vi "Dashboard Main.vi"() -> ()   [LabVIEW 2015]
uses:
  <vilib>/Utility/miscctls.llb/LVRowAndColumnTypeDef.ctl
  <vilib>/event_ctls.llb/eventvkey.ctl
  <vilib>/Rock Robotics/WPI/Dashboard/WPI_DashboardLogging Global.vi
  <vilib>/Rock Robotics/Network Tables/NT Read Numeric Array.vi
  <vilib>/Rock Robotics/Network Tables/NT Write Boolean Array.vi
  <vilib>/Rock Robotics/Network Tables/NT Write Numeric Array.vi
  <vilib>/Rock Robotics/Network Tables/NT Read Boolean Array.vi
  <vilib>/Rock Robotics/Network Tables/NT Write Boolean.vi
  <vilib>/Utility/config.llb/Write Key (String).vi
  <vilib>/Utility/config.llb/Write Key (I32).vi
  <vilib>/Utility/config.llb/NI_LVConfig.lvlib
panel:
  in  "TCP":refnum<k5>
  out "Camera IP":string
  out "Image Message":string="Timeout in Camera Communications"
  in  "Dashboard Tab":T1(tab)
  in  "Select Auto":string(combo)
  out "NT Connection":bool
  in  "Camera Settings":T2={"Frame Rate"=30, "Compression"=30, "Size"=1} {"Frame Rate" scale=1.0..30.0; "Size" items=["640x480", "320x240", "160x120"]}
  out "MotorChart R":cluster{"Numeric":dbl, "Numeric":dbl}(graph)
  out "MotorChart L":T3(graph)
  out "MotorSliders R":cluster{"MotorSlide1":dbl, "MotorSlide2":dbl} {"MotorSlide2" scale=-1.0..1.0 scale format="%#_2e"; "MotorSlide1" scale=-1.0..1.0 scale format="%#_2e"}
  out "MotorSliders L":T4 {"MotorSlide4 2" scale=0.0..14.0 scale format="%#_2e"; "MotorSlide2" scale=-1.0..1.0 scale format="%#_2e"; "MotorSlide1" scale=-1.0..1.0 scale format="%#_2e"}
  out "Gyro":dbl(knob) scale=0.0..360.0
  out "JS1 Z":dbl(slide) scale=-1.0..1.0 scale format="%#_2e"
  out "JS1 Graph":cluster{"X":dbl, "Y":dbl}[](graph)
  out "JS1 Buttons":T5
  out "JS2 Z":dbl(slide) scale=-1.0..1.0 scale format="%#_2e"
  out "JS2 Graph":cluster{"X":dbl, "Y":dbl}[](graph)
  out "JS2 Buttons":T5
  out "Mode":T6(ring)=enum."Auto Disabled"
  in  "DB Camera Config":bool
  out "fps":dbl format="%#.1g"
  out "Mbps":dbl format="%#.1g"
  out "Mbps LED":bool
  in  "Vision":u16(ring) items=["Camera Off", "USB Camera SW", "USB Camera HW", "IP Camera"]
  in  "Rec Mode":enum32{"Stop", "Record", "Playback"}(radio)
  out "Analogue 3":dbl
  out "Analogue 2":dbl
  out "Analogue 1":dbl
  out "Analogue 0":dbl
  in  "SOLENOID 7":bool
  in  "SOLENOID 6":bool
  in  "SOLENOID 5":bool
  in  "SOLENOID 4":bool
  in  "SOLENOID 3":bool
  in  "SOLENOID 2":bool
  in  "SOLENOID 1":bool
  in  "SOLENOID 0":bool
  in  "Compressor":bool
  in  "RELAY 3":enum16{"Off", "On", "Forward", "Reverse"}(ring)
  in  "RELAY 2":enum16{"Off", "On", "Forward", "Reverse"}(ring)
  in  "RELAY 1":enum16{"Off", "On", "Forward", "Reverse"}(ring)
  in  "RELAY 0":enum16{"Off", "On", "Forward", "Reverse"}(ring)
  out "DIO 9":bool
  out "DIO 8":bool
  out "DIO 7":bool
  out "DIO 6":bool
  out "DIO 5":bool
  out "DIO 4":bool
  out "DIO 3":bool
  out "DIO 2":bool
  out "DIO 1":bool
  out "DIO 0":bool
  in  "Motor 2 Controller":T7(radio)
  in  "Invert Motor 2":bool
  out "Current Motor 2 Type":string
  in  "Select Motor 2 Address":dbl
  in  "Select Motor 2 Type":u16(ring)=101 items=["CAN Jaguar"=0, "Jaguar"=1, "CAN Talon"=2, "Talon (SR)"=3, "Talon SRX"=4, "Victor"=5, "Victor SP"=6, "Null"=101]
  in  "Motor 1 Controller":T7(radio)
  in  "Invert Motor 1":bool
  out "Current Motor 1 Type":string
  in  "Select Motor 1 Address":dbl
  in  "Select Motor 1 Type":u16(ring)=101 items=["CAN Jaguar"=0, "Jaguar"=1, "CAN Talon"=2, "Talon (SR)"=3, "Talon SRX"=4, "Victor"=5, "Victor SP"=6, "Null"=101]
  out "Motor 1":dbl(knob) scale=-1.0..1.0
  in  "Set Motor":bool
  in  "Joystick Deadband":dbl=0.2
  out "Motor 2":dbl(knob) scale=-1.0..1.0
  in  "Test Slider":dbl(slide) scale=0.0..100.0 scale format="%#_3g"
  in  "On/Off":bool caption="Solenoid"
  in  "Test Name":u16(ring) items=["Select the test to run..."]
  in  "Test Tree":string(tree)
  in  "Motor":cluster{"Value":dbl, "Enable":bool} {"Value" scale=-1.0..1.0 scale format="%#_3g"}
  out "Progress":T8 {"Test Progress" scale=0.0..100.0}
  in  "Rev/Fwd":cluster{"Forward":bool, "Reverse":bool}
  in  "Test Ring":u16(ring) items=["Monochrome", "Color"]
  out "Cmd Status":string
  in  "Execute Command":bool
  in  "Command Params":string[][](table)
  in  "Command Selection":i32(listbox)
  in  "CheckList":i32(listbox)
  out "Tree":string(tree)
  out "Camera Image":T9(plugin-control)
  out "Background":bool
  # "Left"
  # "Front"
  # "Right"
  # "Battery"
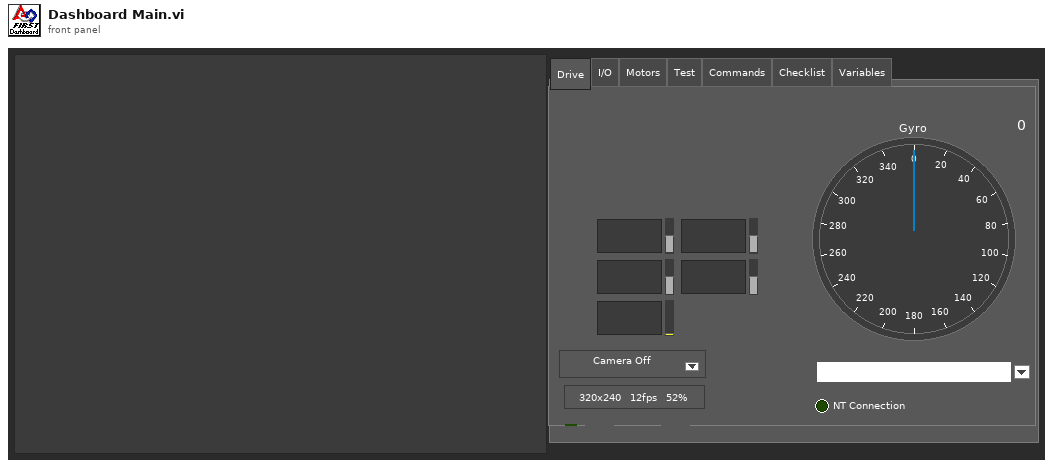
[diagram p1: front panel]
types:
  T1 = enum32{"Drive", "I/O", "Motors", "Test", "Commands", "Checklist", "Variables"}
  T2 = cluster{"Frame Rate":i32, "Compression":i32, "Size":u16}
  T3 = cluster{"Numeric":dbl, "Numeric":dbl, "Battery V":dbl}
  T4 = cluster{"MotorSlide1":dbl, "MotorSlide2":dbl, "MotorSlide4 2":dbl}
  T5 = cluster{bool, bool, bool, bool, bool, bool, bool, bool, bool, bool, bool, bool}
  T6 = enum8{"Tele-Op Disabled", "Tele-Op Enabled", "Auto Disabled", "Auto Enabled", "Test Disabled", "Test Enabled", "Disconnected", "No Code", "E-Stop"}
  T7 = enum32{"Radio Selection 1", "Radio Selection 2", "Radio Selection 3"}
  T8 = cluster{"Test Progress":u8, "Test Progress Text":string}
  T9 = typedef "IMAQ Image.ctl" = refnum<image>
  T10 = cluster{"IDs":cluster{"RPC field ID":u16, "Unique ID":u16}, "String":string}
  T11 = enum32{"Drive", "Basic", "Custom", "Test", "Checklist", "Variables"}
  T12 = typedef "Image Type" = u32
  T13 = cluster{"Camera Image":refnum<vi>, "Dashboard Tab":refnum<vi>, "Background":refnum<vi>, "Vision":refnum<vi>, "Rec Mode":refnum<vi>, "Test Slider":refnum<vi>, "On/Off ":refnum<vi>, "Test Ring":refnum<vi>, "Rev/Fwd":refnum<vi>, "Test Name":refnum<vi>, "Motor":refnum<vi>, "Progress":refnum<vi>, "CheckList":refnum<vi>, "Tree":refnum<vi>, "Test Tree":refnum<vi>, "Command Params":refnum<vi>, "Command Selection":refnum<vi>, "Execute Command":refnum<vi>, "Cmd Status":refnum<vi>}
  T14 = cluster{"Error Strings":string, "Disable Counts":cluster{u16, u16}, "Rail Faults":cluster{u16, u16, u16}, "Robot IP":string, "DB Mode":u8, "Event Info":cluster{"Name":string, "Type":u8, "Number":u16, "Replay":u8}, "Camera Addr":string}
  T15 = cluster{"Storage":cluster{"Disk Free":u64, "RAM Block":u32, "RAM free":u32}, "CPU Utilization":cluster{"CPU % ISR":sgl, "CPU % Time Crit":sgl, "CPU % Timed Str":sgl, "CPU % High":sgl, "CPU % Above":sgl, "CPU % Normal":sgl, "CPU % Low":sgl}, "CAN":cluster{"% Bus Utilization":sgl, "Bus Off Cnt":u32, "TX_FIFO Full Cnt":u32, "Receive Error Cnt":u8, "Transmit Error Cnt":u8}, "HID":cluster{"HID Outputs":u32, "Rumble Low":u16, "Rumble High":u16}[]}
  T16 = cluster{"Status bits":cluster{"Test Mode":bool, "Autonomous":bool, "Enabled":bool, "Code Start":bool, "Brownout":bool, "Reserved 2":bool, "Reserved 3":bool, "E-Stop":bool}, "Code Trace":cluster{"Disabled":bool, "TeleOp":bool, "Auto":bool, "Test":bool}, "Controller Type":enum16{"unknown", "cRIO", "roboRio"}, "Code?":enum16{"unknown", "noCode", "code"}, "Battery V":dbl}
  T17 = cluster{"Control Bits":cluster{"TestMode":bool, "Autonomous":bool, "Enabled":bool, "FMS Present":bool, bool, bool, bool, "E-Stop":bool}, "Team Station ":u8, "Countdown":sgl, "Joystick Values":cluster{"Axes":dbl[], "Buttons":bool[], "POVs":i16[]}[]}
  T18 = cluster{"Axes":dbl[], "Buttons":bool[], "POVs":i16[]}[]
  T19 = cluster{"Axes":dbl[], "Buttons":bool[], "POVs":i16[]}
  T20 = cluster{"Buttons[0]":bool, "Buttons[1]":bool, "Buttons[2]":bool, "Buttons[3]":bool, "Buttons[4]":bool, "Buttons[5]":bool, "Buttons[6]":bool, "Buttons[7]":bool, "Buttons[8]":bool, "Buttons[9]":bool, "Buttons[10]":bool, "Buttons[11]":bool}
  T21 = typedef "NI_LVConfig.lvlib/Config Data RefNum.ctl" = refnum<k1>
  T22 = cluster{"Operation":enum16{"Update", "Clear"}, "Color Box":u32}[]
  T23 = typedef "eventvkey.ctl" = enum16{"ASCII", "Enter", "Return", "Shift", "Ctrl", "Alt", "Cmd", "Opt", "Caps", "NumLock", "Clear", "Break", "Up", "Down", "Left", "Right", "Insert", "Delete", "Home", "End", "PageUp", "PageDown", "Escape", "Help", "Pause", "ScrollLock", "F1", "F2", "F3", "F4", "F5", "F6", "F7", "F8", "F9", "F10", "F11", "F12", "F13", "F14", "F15", "F16", "F17", "F18", "F19", "F20", "F21", "F22", "F23", "F24", "Play", "VolumeUp", "VolumeDown", "Mute", "Two Byte Char"}
  T24 = cluster{"Image Size":bool, "Image Type":bool, "Pixel Value":bool, "ROI Information":bool, "Zoom Factor":bool}
  T25 = enum8{"Enabled", "Disabled", "Disabled and Grayed Out"}
  T26 = cluster{"Operation":enum16{"Update", "Clear"}, "Color Box":u32}
  T27 = typedef "LVRowAndColumnTypeDef.ctl" = cluster{"Row":i32, "Column":i32}
  T28 = cluster{"Shift":bool, "Ctrl":bool, "Alt":bool, "Cmd":bool, "Opt":bool}
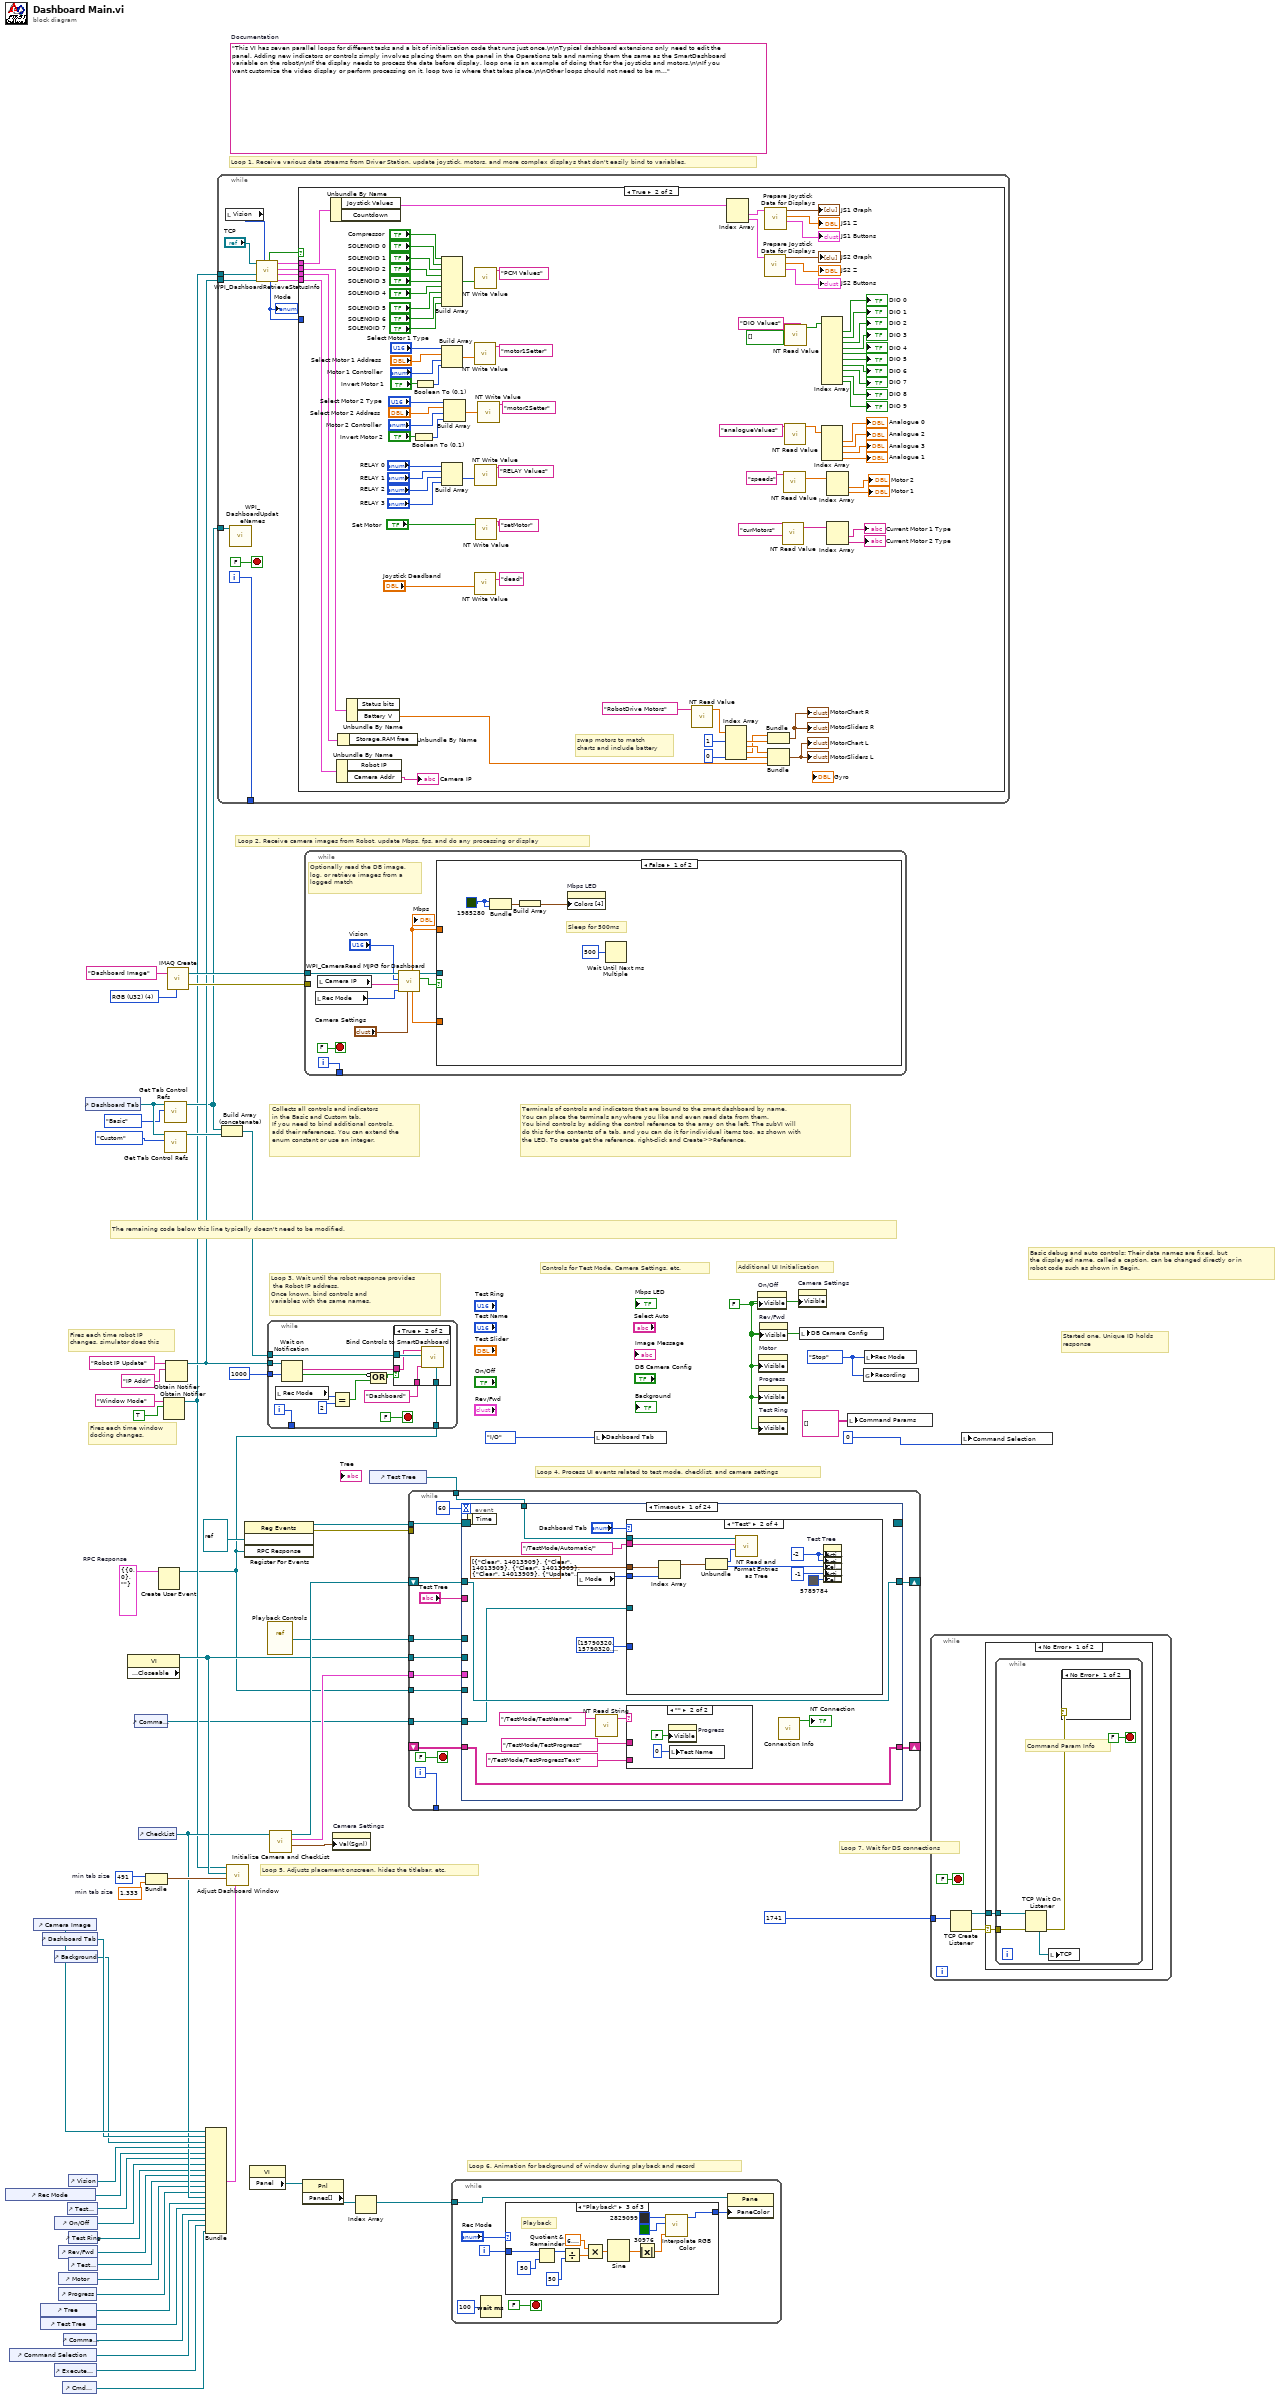
[diagram p0: block diagram]
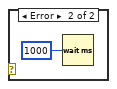
[diagram p2: hidden frame]
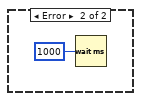
[diagram p3: hidden frame]
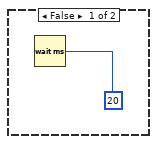
[diagram p4: hidden frame]
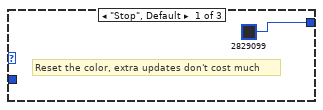
[diagram p5: hidden frame]
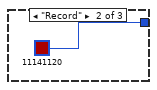
[diagram p6: hidden frame]
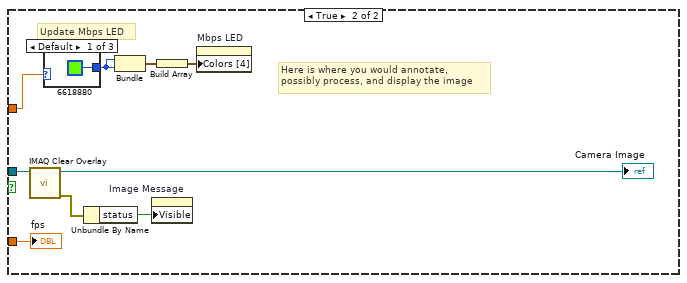
[diagram p8: hidden frame]
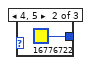
[diagram p9: hidden frame]
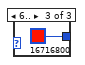
[diagram p10: hidden frame]
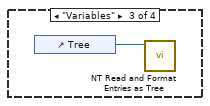
[diagram p12: hidden frame]
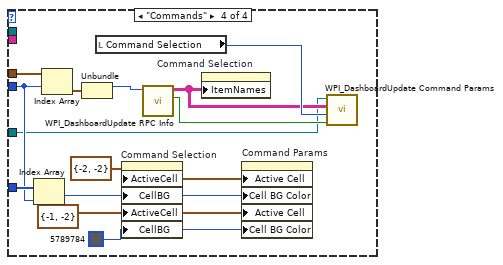
[diagram p13: hidden frame]
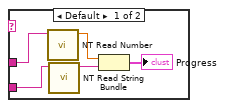
[diagram p14: hidden frame]
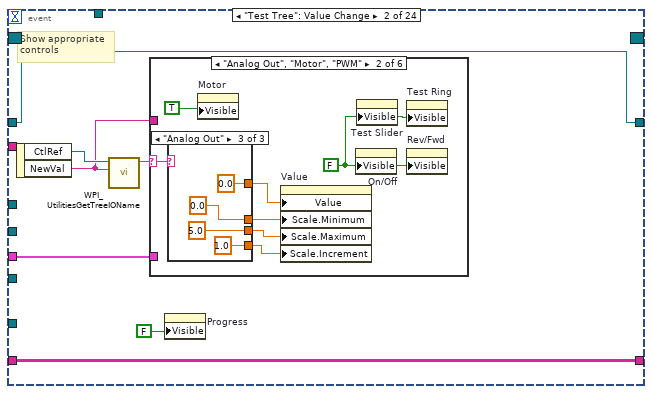
[diagram p15: hidden frame]
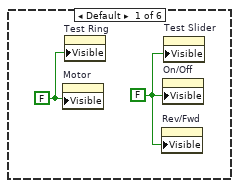
[diagram p16: hidden frame]
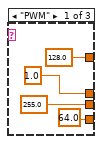
[diagram p17: hidden frame]
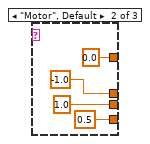
[diagram p18: hidden frame]
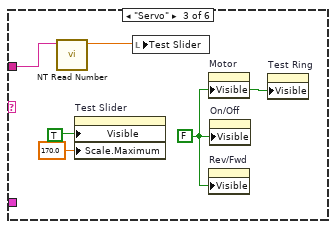
[diagram p19: hidden frame]
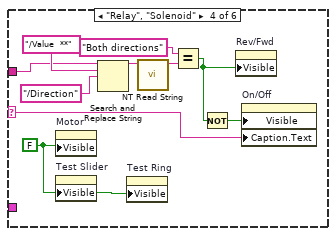
[diagram p20: hidden frame]
diagram:
  w7 = T10 {"IDs"={"RPC field ID"=0, "Unique ID"=0}, "String"=""}  # RPC Response
  w33 = 491  # min tab size
  w32 = 1.333  # min tab size
  w41 = enum32{"Stop", "Record", "Playback"}."Stop" ("Rec Mode")
  w15 = FALSE ("Visible")
  (unwired) "This VI has seven parallel loops for different tasks and a bit of initialization code that runs just once.\n\nTypical dashboard extensions only need to edit the panel. Adding new indicators or controls simply involves placing them on the panel in the Operations tab and naming them the same as the SmartDashboard variable on the robot\n\nIf the display needs to process the data before display, loop one is an example of doing that for the joysticks and motors.\n\nIf you want customize the video display or perform processing on it, loop two is where that takes place.\n\nOther loops should not need to be modified. They are pretty standard, and document the task they perform."  # Documentation
  w61 = T12 4 items=["Grayscale (U8)", "Grayscale (I16)", "Grayscale (SGL)", "Complex (CSG)", "RGB (U32)", "HSL (U32)", "RGB (U64)"] ("Image Type")
  # "Command Param Info"
  # "Started one, Unique ID holds\nresponse"
  # "Loop 7. Wait for DS connections"
  # "Basic debug and auto controls: Their data names are fixed, but\nthe displayed name, called a caption, can be changed directly or in\nrobot code such as shown in Begin."
  # "Controls for Test Mode, Camera Settings, etc."
  # "Additional UI Initialization"
  # "Loop 6. Animation for background of window during playback and record"
  # "Fires each time robot IP\nchanges, simulator does this"
  # "Fires each time window\ndocking changes."
  # "Collects all controls and indicators\nin the Basic and Custom tab.\nIf you need to bind additional controls,\nadd their references. You can extend the\nenum constant or use an integer."
  # "The remaining code below this line typically doesn't need to be modified."
  # "Loop 4. Process UI events related to test mode, checklist, and camera settings"
  # "Terminals of controls and indicators that are bound to the smart dashboard by name.\nYou can place the terminals anywhere you like and even read data from them.\nYou bind controls by adding the control reference to the array on the left. The subVI will\ndo this for the contents of a tab, and you can do it for individual items too, as shown with\nthe LED. To create get the reference, right-click and Create>>Reference."
  # "Loop 3. Wait until the robot response provides\n the Robot IP address.\nOnce known, bind controls and\nvariables with the same names."
  # "Loop 5. Adjusts placement onscreen, hides the titlebar, etc."
  # "Loop 1. Receive various data streams from Driver Station, update joystick, motors, and more complex displays that don't easily bind to variables."
  # "Loop 2. Receive camera images from Robot, update Mbps, fps, and do any processing or display"
  n1 = control-ref of="Rec Mode"() -> (w21:refnum<vi>)
  n2 = control-ref of="Command Selection"() -> (w6:refnum<vi>)
  n3 = control-ref of="Camera Image"() -> (w36:refnum<vi>)
  n4 = control-ref of="Tree"() -> (w25:refnum<vi>)
  n5 = control-ref of="Test Tree"() -> (w24:refnum<vi>)
  n6 = control-ref of="Dashboard Tab"() -> (w35:refnum<vi>)
  n7 = control-ref of="Execute Command"() -> (w8:refnum<vi>)
  n8 = control-ref of="Background"() -> (w30:refnum<vi>)
  n9 = control-ref of="On/Off"() -> (w19:refnum<vi>)
  n10 = control-ref of="Progress"() -> (w16:refnum<vi>)
  n11 = control-ref of="Rev/Fwd"() -> (w17:refnum<vi>)
  n12 = control-ref of="Motor"() -> (w22:refnum<vi>)
  n13 = control-ref of="Cmd Status"() -> (w2:refnum<vi>)
  n14 = control-ref of="Command Params"() -> (w9:refnum<vi>)
  n15 = control-ref of="Test Slider"() -> (w20:refnum<vi>)
  n16 = control-ref of="Vision"() -> (w34:refnum<vi>)
  n17 = control-ref of="Test Ring"() -> (w18:refnum<vi>)
  n18 = control-ref of="Test Name"() -> (w23:refnum<vi>)
  n19 = control-ref of="Dashboard Tab"() -> (w39:refnum<vi>)
  n20 = property class="VI" props=["Front Panel.Closeable"]() -> (reference out=w40:refnum<vi>)  [unwired: 2 in, 2 out]
  n21 = control-ref of="Command Params"() -> (w1:refnum<vi>)
  n22 = control-ref of="CheckList"() -> (w26:refnum<vi>)
  n23 = Bundle("min tab size"=w33, "min tab size"=w32) -> (w31:cluster{"min tab size":i32, "min tab size":dbl})  [unwired: 1 in]
  n24 = Create User Event(user event datatype=w7) -> (user event=w3:refnum<user-event>)  [unwired: 1 in, 1 out]
  n25 = Obtain Notifier(name (unnamed)="Window Mode", notification data type=TRUE) -> (notifier out=w12:refnum<notifier>)  [unwired: 2 in, 2 out]
  n26 = call <vilib>:"Get Tab Control Refs.vi"("Page Index"=T11."Basic" ("Dashboard Tab"), "TabControl in"=w39) -> ("ControlsOnPage"=w13:refnum<vi>[])  [unwired: 9 in]
  n27 = call <vilib>:"Get Tab Control Refs.vi"("Page Index"=T11."Custom" ("Dashboard Tab"), "TabControl in"=w39) -> ("ControlsOnPage"=w38:refnum<vi>[])  [unwired: 9 in]
  n28 = Obtain Notifier(name (unnamed)="Robot IP Update", notification data type="IP Addr" ("name (unnamed)")) -> (notifier out=w14:refnum<notifier>)  [unwired: 2 in, 2 out]
  n29 = call "IMAQ Create"("Image Name"="Dashboard Image", "Image Type"=w61) -> ("New Image"=w59:T9, "error out"=w58:errorcluster)  [unwired: 2 in, 1 out]
  n30 = Bundle("Camera Image"=w36, "Dashboard Tab"=w35, "Background"=w30, "Vision"=w34, "Rec Mode"=w21, "Test Slider"=w20, "On/Off"=w19, "Test Ring"=w18, "Rev/Fwd"=w17, "Test Name"=w23, "Motor"=w22, "Progress"=w16, "CheckList"=w26, "Tree"=w25, "Test Tree"=w24, "Command Params"=w9, "Command Selection"=w6, "Execute Command"=w8, "Cmd Status"=w2) -> (w27:T13)  [unwired: 1 in]
  n31 = while {
    tunnel: [w73] -> _
    tunnel: w14 -> [w67]
    tunnel: w13 -> [w66]
    tunnel: w12 -> [w62]
    i -> [w73]
    stop <- FALSE stop-if-true
    n32 = local read "Vision"() -> (w64:u16)
    n33 = call <vilib>:"WPI_DashboardUpdateNames.vi"("Controls on Tab"=w66) -> ()  [unwired: 11 in]
    n34 = call <vilib>:"WPI_DashboardRetrieveStatusInfo.vi"("Vision"=w64, "Binding Refnum"=w67, "Window Mode Notifier"=w62, "TCP Cnx"="TCP") -> ("Power and Errors"=w68:T14, "Robot Metrics"=w71:T15, "Status Info"=w72:T16, "Control Info"=w69:T17, "Robot Mode"=w65:T6, "Process?"=w70:bool)  [unwired: 2 in]
    "Mode" <- w65
    n35 = case shown="True" w70 {
      tunnel: w72 -> [_ w162]
      tunnel: w71 -> [_ w161]
      tunnel: w69 -> [_ w160]
      tunnel: w68 -> [_ w159]
      tunnel: w65 -> [_ _]
      frame False {
        n36 = Wait (ms)(milliseconds to wait=u32 20) -> ()  [unwired: 1 out]
      }
      frame True {
        # "swap motors to match\ncharts and include battery"
        n37 = Unbundle By Name(w160) -> ("Joystick Values"=w149:T18)  [unwired: 1 out]
        n38 = Unbundle By Name(w159) -> ("Camera Addr"=→"Camera IP":string)  [unwired: 1 out]
        n39 = Unbundle By Name(w161) -> ()  [unwired: 1 out]
        n40 = Unbundle By Name(w162) -> ("Battery V"=w150:dbl)  [unwired: 1 out]
        n41 = Boolean To (0,1)(Boolean="Invert Motor 2") -> (0, 1=w80:i16)
        n42 = Boolean To (0,1)(Boolean="Invert Motor 1") -> (0, 1=w92:i16)
        n43 = Build Array("Compressor", "SOLENOID 0", "SOLENOID 1", "SOLENOID 2", "SOLENOID 3", "SOLENOID 4", "SOLENOID 5", "SOLENOID 6", "SOLENOID 7") -> (w124:bool[])
        n44 = Build Array("Select Motor 1 Type", "Select Motor 1 Address", "Motor 1 Controller", w92) -> (w108:dbl[])
        n45 = Build Array("RELAY 0", "RELAY 1", "RELAY 2", "RELAY 3") -> (w115:enum16{"Off", "On", "Forward", "Reverse"}[])
        n46 = Build Array("Select Motor 2 Type", "Select Motor 2 Address", "Motor 2 Controller", w80) -> (w79:dbl[])
        n47 = call-poly <vilib>:"NT Write Value.vi"("Numeric Array"=w108, "Name"="motor1Setter") -> ()  [unwired: 9 in, 1 out]
        n48 = call-poly <vilib>:"NT Write Value.vi"("Numeric"="Joystick Deadband", "Name"="dead") -> ()  [unwired: 9 in, 1 out]
        n49 = call-poly <vilib>:"NT Write Value.vi"("Boolean Array"=w124, "Name"="PCM Values") -> ()  [unwired: 9 in, 1 out]
        n50 = call-poly <vilib>:"NT Write Value.vi"("Numeric Array"=w115, "Name"="RELAY Values") -> ()  [unwired: 9 in, 1 out]
        n51 = call-poly <vilib>:"NT Write Value.vi"("Boolean"="Set Motor", "Name"="setMotor") -> ()  [unwired: 9 in, 1 out]
        n52 = call-poly <vilib>:"NT Write Value.vi"("Numeric Array"=w79, "Name"="motor2Setter") -> ()  [unwired: 9 in, 1 out]
        n53 = call-poly <vilib>:"NT Read Value.vi"("Name"="RobotDrive Motors") -> ("Numeric Array"=w138:dbl[])  [unwired: 9 in, 1 out]
        n54 = Index Array(array=w138, index #1=1, index #4=0) -> (element #1=w154:dbl, element #2=w155:dbl, element #3=w153:dbl, element #4=w158:dbl)  [unwired: 2 in]
        n55 = Index Array(array=w149) -> (element #1=w148:T19, element #2=w143:T19)  [unwired: 2 in]
        n56 = call "Prepare Joystick Data for Displays.vi"("Joystick Values"=w143) -> ("Buttons"=→"JS2 Buttons":T20, "Z Axis"=→"JS2 Z":dbl, "Cartesian Data"=→"JS2 Graph":cluster{"X axis":dbl, "X axis":dbl}[])  [unwired: 8 in]
        n57 = call "Prepare Joystick Data for Displays.vi"("Joystick Values"=w148) -> ("Buttons"=→"JS1 Buttons":T20, "Z Axis"=→"JS1 Z":dbl, "Cartesian Data"=→"JS1 Graph":cluster{"X axis":dbl, "X axis":dbl}[])  [unwired: 8 in]
        n58 = Bundle("Numeric"=w153, "Numeric"=w154) -> (→"MotorChart R" →"MotorSliders R":cluster{"Numeric":dbl, "Numeric":dbl})  [unwired: 1 in]
        n59 = Bundle("Numeric"=w155, "Numeric"=w158, "Battery V"=w150) -> (→"MotorChart L" →"MotorSliders L":T3)  [unwired: 1 in]
        n60 = call-poly <vilib>:"NT Read Value.vi"("Name"="curMotors") -> ("String Array"=w87:string[])  [unwired: 9 in, 1 out]
        n61 = call-poly <vilib>:"NT Read Value.vi"("Name"="speeds") -> ("Numeric Array"=w91:dbl[])  [unwired: 9 in, 1 out]
        n62 = call-poly <vilib>:"NT Read Value.vi"("Name"="analogueValues") -> ("Numeric Array"=w104:dbl[])  [unwired: 9 in, 1 out]
        n63 = call-poly <vilib>:"NT Read Value.vi"("Default Value"=bool[] [], "Name"="DIO Values") -> ("Boolean Array"=w137:bool[])  [unwired: 8 in, 1 out]
        n64 = Index Array(array=w137) -> (element #1=→"DIO 0":bool, element #2=→"DIO 1":bool, element #3=→"DIO 2":bool, element #4=→"DIO 3":bool, element #5=→"DIO 4":bool, element #6=→"DIO 5":bool, element #7=→"DIO 6":bool, element #8=→"DIO 7":bool, element #9=→"DIO 8":bool, element #10=→"DIO 9":bool)  [unwired: 10 in]
        n65 = Index Array(array=w104) -> (element #1=→"Analogue 0":dbl, element #2=→"Analogue 2":dbl, element #3=→"Analogue 3":dbl, element #4=→"Analogue 1":dbl)  [unwired: 4 in]
        n66 = Index Array(array=w91) -> (element #1=→"Motor 2":dbl, element #2=→"Motor 1":dbl)  [unwired: 2 in]
        n67 = Index Array(array=w87) -> (element #1=→"Current Motor 1 Type":string, element #2=→"Current Motor 2 Type":string)  [unwired: 2 in]
      }
    }
  }
  n68 = Build Array (concatenate)(w13, w38) -> (w37:refnum<vi>[])
  n69 = call "Adjust Dashboard Window.vi"("Sizing Refnums"=w27, "Size Constraints"=w31, "VI"=w40, "WIn Mode"=w12) -> ()  [unwired: 8 in]
  n70 = register-events(refnum<vi> refnum, w3) -> (reference out=w45:refnum<event-registration>, error out=w44:errorcluster)  [unwired: 2 in]
  n71 = property class="VI"() -> ("Panel"=w48:refnum<vi>)  [unwired: 2 in, 2 out]
  n72 = while {
    tunnel: w37 -> [w175]
    tunnel: w14 -> [w173]
    tunnel: [w171] -> _
    tunnel: u32 1000 ("milliseconds to wait") -> [w170]
    tunnel: w3 -> [w163]
    i -> [w171]
    stop <- FALSE stop-if-true
    n73 = local read "Rec Mode"() -> (w166:enum32{"Stop", "Record", "Playback"})
    n74 = Wait on Notification(notifier=w173, timeout in ms (-1)=w170) -> (notification=w172:string, timed out?=w168:bool)  [unwired: 2 in, 2 out]
    n75 = Equal?(x=w166, y=u16 2 ("Rec Mode")) -> (x = y?=w167:bool)
    n76 = Compound Arithmetic op=OR(invert w168, w167) -> (w169:bool)
    n77 = case shown="True" w169 {
      tunnel: w175 -> [_ w179]
      tunnel: w172 -> [_ w178]
      tunnel: "Dashboard" -> [_ w177]
      tunnel: w163 -> [_ w176]
      frame False {
      }
      frame True {
        n78 = call <vilib>:"Bind Controls to SmartDashboard.vi"("RPC ref"=w176, "Client Name"=w177, "Bound Control Refs"=w179, "Server IP Address"=w178) -> ()  [unwired: 8 in]
      }
    }
  }
  n79 = vi-ref "Playback Controls.vi"() -> (w46:refnum<vi>)
  n80 = call "Initialize Camera and CheckList.vi"("ListBox in"=w26) -> ("Cluster"=w52:cluster{"value":i32, "value":i32, "index":i32}, "Array"=w53:cluster{string[]}[], "File Refnum"=w51:T21)  [unwired: 8 in]
  n81 = property class="Pnl"(reference=w48) -> ("Panes[]"=w49:refnum<vi>[])  [unwired: 1 in, 2 out]
  n82 = while {
    tunnel: w59 -> [w188]
    tunnel: w58 -> [_]
    tunnel: [w189] -> _
    i -> [w189]
    stop <- FALSE stop-if-true
    # "Optionally read the DB image,\nlog, or retrieve images from a\nlogged match"
    n83 = local read "Rec Mode"() -> (w183:enum32{"Stop", "Record", "Playback"})
    n84 = local read "Camera IP"() -> (w181:string)
    n85 = call <vilib>:"WPI_CameraRead MJPG for Dashboard.vi"("Camera Settings"="Camera Settings", "Rec Mode"=w183, "Camera IP"=w181, "Camera Mode"="Vision", "Refnum in"=w188) -> ("Active"=w186:bool, "Refnum out"=w187:T9, "FPS"=w185:dbl, "Bandwidth (Mbps)"=w180:dbl)  [unwired: 3 in]
    "Mbps" <- w180
    n86 = case shown="False" w186 {
      tunnel: w187 -> [_ w198]
      tunnel: w180 -> [_ w197]
      tunnel: w185 -> [_ w195]
      frame False {
        w191 = u32 1985280 ("Color Box")
        # "Sleep for 500ms"
        n87 = Bundle("Color Box"=w191, "Color Box"=w191) -> (w193:cluster{"Color Box":u32, "Color Box":u32})  [unwired: 1 out]
        n88 = Build Array(w193) -> (w192:cluster{"Color Box":u32, "Color Box":u32}[])
        n89 = property on="Mbps LED" class="Bool (strict)"("Colors [4]"=w192) -> ()  [unwired: 2 in, 2 out]
        n90 = Wait Until Next ms Multiple(millisecond multiple=u32 500) -> ()  [unwired: 1 out]
      }
      frame True {
        # "Here is where you would annotate,\npossibly process, and display the image"
        # "Update Mbps LED"
        n91 = call "IMAQ Clear Overlay"("Image"=w198) -> ("error out"=w202:errorcluster, "Image Out"=→"Camera Image":T9)  [unwired: 2 in, 7 out]
        n92 = case shown="Default" w197 {
          tunnel: [u32 6618880 ("Color Box") u32 16776722 ("Color Box") u32 16716800 ("Color Box")] -> w199
          frame Default {
          }
          frame 4, 5 {
          }
          frame 6.. {
          }
        }
        n93 = Unbundle By Name(w202) -> ("status"=w203:bool)
        n94 = Bundle("Color Box"=w199, "Color Box"=w199) -> (w201:cluster{"Color Box":u32, "Color Box":u32})  [unwired: 1 out]
        n95 = property on="Image Message" class="Str"("Visible"=w203) -> ()  [unwired: 2 in, 2 out]
        n96 = Build Array(w201) -> (w200:cluster{"Color Box":u32, "Color Box":u32}[])
        n97 = property on="Mbps LED" class="Bool (strict)"("Colors [4]"=w200) -> ()  [unwired: 2 in, 2 out]
        "fps" <- w195
      }
    }
  }
  n98 = property on="Camera Settings" class="Clust (strict)"("Val(Sgnl)"=w52) -> ()  [unwired: 2 in, 2 out]
  n99 = Index Array(array=w49) -> (element=w47:refnum<vi>)  [unwired: 1 in]
  n100 = control-ref of="Test Tree"() -> (w50:refnum<vi>)
  n101 = while {
    tunnel: w53 -> [w218]
    shift-right: [w217] -> _
    shift-left: w51 -> [w216]
    tunnel: [w215] -> _
    tunnel: w50 -> [w214]
    tunnel: w46 -> [w213]
    tunnel: w45 -> [w212]
    tunnel: w44 -> [_]
    tunnel: w40 -> [w211]
    tunnel: w3 -> [w210]
    tunnel: w1 -> [w209]
    shift-right: [w208] -> _
    shift-left: _ -> [w207]
    i -> [w215]
    stop <- FALSE stop-if-true
    n102 = event shown="[0] Timeout" {
      selector: w212 -> [_ _ _ _ _ _ _ _ _ _ _ _ _ _ _ _ _ _ _ _ _ _ _ _]
      dyn-events: [_ _ _ _ _ _ _ _ _ _ _ _ _ _ _ _ _ _ w527 _ _ _ _ _] -> _
      timeout: u32 60 ("milliseconds to wait") -> [_ _ _ _ _ _ _ _ _ _ _ _ _ _ _ _ _ _ _ _ _ _ _ _]
      tunnel: w214 -> [w231 _ _ _ _ _ _ _ _ _ _ _ _ _ _ _ _ _ _ _ _ _ _ _]
      tunnel: "Test Tree" -> [_ _ _ _ _ _ _ _ _ _ _ _ _ w490 w499 w502 w507 w516 _ _ _ _ _ _]
      tunnel: w218 -> [_ w269 _ _ _ _ _ _ _ _ _ w452 w483 _ _ _ _ _ _ _ _ _ _ _]
      tunnel: [w228 w268 w372 w378 w388 w392 w398 w410 w418 w424 w437 w451 w476 w489 w497 w501 w506 w515 w529 w545 w547 w555 w566 w571] -> w217
      tunnel: w216 -> [w228 w268 w372 w378 w388 w392 w398 w410 w418 w424 w437 w450 w476 w489 w497 w501 w506 w515 w529 w545 w547 w555 w566 w571]
      tunnel: w213 -> [_ _ _ _ _ _ _ _ _ _ _ _ _ _ _ _ _ _ w530 _ w550 _ _ _]
      tunnel: w211 -> [_ _ _ _ _ _ _ _ _ _ _ _ _ _ _ _ _ _ w525 _ _ _ _ _]
      tunnel: w210 -> [_ _ _ _ _ _ _ _ _ _ _ _ _ _ _ _ _ _ w521 _ _ _ _ _]
      tunnel: w209 -> [w223 _ _ _ _ _ w396 _ _ _ _ _ _ _ _ _ _ _ _ _ _ _ _ _]
      tunnel: [w222 w267 w371 w377 w387 w393 w394 w404 w415 w423 w436 w449 w475 w488 w496 w500 w505 w514 w520 w543 w546 w551 w559 w572] -> w208
      tunnel: w207 -> [w222 w267 w371 w377 w387 w393 w394 _ _ w423 w436 w449 w475 w488 w496 w500 w505 w514 w520 w543 w546 w551 w559 w572]
      event Timeout {
        n103 = event-data() -> ()  [unwired: 1 in, 1 out]
        n104 = local read "Mode"() -> (w225:T6)
        n105 = call <vilib>:"NT Read String.vi"("Name"="/TestMode/TestName") -> ("String"=w234:string)  [unwired: 9 in, 1 out]
        n106 = case shown="\"Test\"" "Dashboard Tab" {
          tunnel: w231 -> [_ w245 _ _]
          tunnel: "/TestMode/Automatic/" ("Name Pattern") -> [_ w244 _ _]
          tunnel: T22 [{"Operation"=enum."Clear", "Color Box"=14013909}, {"Operation"=enum."Clear", "Color Box"=14013909}, {"Operation"=enum."Clear", "Color Box"=14013909}, {"Operation"=enum."Clear", "Color Box"=14013909}, {"Operation"=enum."Update", "Color Box"=14013909}, {"Operation"=enum."Update", "Color Box"=16777215}, {"Operation"=enum."Clear", "Color Box"=14013909}, {"Operation"=enum."Clear", "Color Box"=14013909}, {"Operation"=enum."Clear", "Color Box"=14013909}] -> [_ w237 _ w254]
          tunnel: w225 -> [_ w236 _ w253]
          tunnel: u32[] [15790320, 15790320, 15790320, 15790320, 16777215, 16777215, 15790320, 15790320, 15790320] -> [_ _ _ w259]
          tunnel: w223 -> [_ _ _ w247]
          frame "I/O", Default {
          }
          frame "Test" {
            w243 = -2 ("Active Item:Row Number")
            n107 = Index Array(array=w237, index=w236) -> (element=w238:T26)
            n108 = Unbundle(w238) -> ("Operation"=w239:enum16{"Update", "Clear"}, "Color Box"=w240:u32)
            n109 = call <vilib>:"NT Read and Format Entries as Tree.vi"("Operation"=w239, "Name Pattern"=w244, "Tree Refnum"=w245) -> ()  [unwired: 7 in, 2 out]
            n110 = property on="Test Tree" class="Tree (strict)"("Active Item Row Number"=w243, "ActiveColNum"=w243, "CellBG"=w240, "Active Item Row Number"=-1 ("Active Item:Row Number"), "CellBG"=u32 5789784 ("Color Box")) -> ()  [unwired: 2 in, 2 out]
          }
          frame "Variables" {
            n111 = control-ref of="Tree"() -> (w246:refnum<vi>)
            n112 = call <vilib>:"NT Read and Format Entries as Tree.vi"("Tree Refnum"=w246) -> ()  [unwired: 9 in, 2 out]
          }
          frame "Commands" {
            w255 = u32 5789784 ("Color Box")
            w256 = T27 {"Row"=-1, "Column"=-2} ("Active Cell:Active Cell")
            w258 = T27 {"Row"=-2, "Column"=-2} ("Active Cell:Active Cell")
            n113 = Index Array(array=w259, index=w253) -> (element=w257:u32)
            n114 = Index Array(array=w254, index=w253) -> (element=w252:T26)
            n115 = Unbundle(w252) -> ("Operation"=w251:enum16{"Update", "Clear"})  [unwired: 1 out]
            n116 = local read "Command Selection"() -> (w250:i32)
            n117 = property on="Command Selection" class="MCListbox (strict)"("ActiveCell"=w258, "CellBG"=w257, "ActiveCell"=w256, "CellBG"=w255) -> ()  [unwired: 2 in, 2 out]
            n118 = call <vilib>:"WPI_DashboardUpdate RPC Info.vi"("Operation"=w251) -> ("update"=w249:bool, "commands"=w248:string[][])  [unwired: 9 in]
            n119 = property on="Command Selection" class="MCListbox (strict)"("ItemNames"=w248) -> ()  [unwired: 2 in, 2 out]
            n120 = property on="Command Params" class="Tbl (strict)"("Active Cell"=w258, "Cell BG Color"=w257, "Active Cell"=w256, "Cell BG Color"=w255) -> ()  [unwired: 2 in, 2 out]
            n121 = call <vilib>:"WPI_DashboardUpdate Command Params.vi"("Update"=w249, "NewVal"=w250, "Commands"=w248, "Param Tbl"=w247) -> ()  [unwired: 7 in, 1 out]
          }
        }
        n122 = case shown="\"\"" w234 {
          tunnel: "/TestMode/TestProgress" ("Name") -> [w261 _]
          tunnel: "/TestMode/TestProgressText" ("Name") -> [w260 _]
          frame Default {
            n123 = call <vilib>:"NT Read Number.vi"("Name"=w261) -> ("Numeric"=w262:dbl)  [unwired: 9 in, 1 out]
            n124 = call <vilib>:"NT Read String.vi"("Name"=w260) -> ("String"=w263:string)  [unwired: 9 in, 1 out]
            n125 = Bundle("Numeric"=w262, "String"=w263) -> (→"Progress":cluster{"Numeric":dbl, "String":string})  [unwired: 1 in]
          }
          frame "" {
            n126 = property on="Progress" class="Clust (strict)"("Visible"=FALSE) -> ()  [unwired: 2 in, 2 out]
            n127 = local write "Test Name"(u16 0) -> ()
          }
        }
        n128 = call <vilib>:"Connextion Info.vi"() -> ("Connected"=→"NT Connection":bool)  [unwired: 10 in, 1 out]
      }
      event "Test Tree": Value Change {
        # "Show appropriate\ncontrols"
        n129 = event-data() -> ("CtlRef"=w272:refnum<vi>, "NewVal"=w270:string)  [unwired: 1 in]
        n130 = call <vilib>:"WPI_UtilitiesGetTreeIOName.vi"("NewVal"=w270, "TreeControl in"=w272) -> ("I/O Name"=w273:string)  [unwired: 9 in]
        n131 = case shown="\"Analog Out\", \"Motor\", \"PWM\"" w273 {
          selector: w273 -> [_ w280 _ w302 w311 _]
          tunnel: w270 -> [_ _ w299 w301 _ w318]
          tunnel: w269 -> [_ _ _ _ _ w317]
          frame Default {
            w275 = FALSE ("Visible")
            w274 = FALSE ("Visible")
            n132 = property on="Motor" class="Clust (strict)"("Visible"=w274) -> ()  [unwired: 2 in, 2 out]
            n133 = property on="Test Ring" class="Ring (strict)"("Visible"=w274) -> ()  [unwired: 2 in, 2 out]
            n134 = property on="Rev/Fwd" class="Clust (strict)"("Visible"=w275) -> ()  [unwired: 2 in, 2 out]
            n135 = property on="On/Off" class="Bool (strict)"("Visible"=w275) -> ()  [unwired: 2 in, 2 out]
            n136 = property on="Test Slider" class="Slide (strict)"("Visible"=w275) -> ()  [unwired: 2 in, 2 out]
          }
          frame "Analog Out", "Motor", "PWM" {
            w281 = FALSE ("Visible")
            n137 = case shown="\"Analog Out\"" w280 {
              tunnel: [1.0 ("Value") -1.0 ("Value") 0.0 ("Value")] -> w279
              tunnel: [255.0 ("Value") 1.0 ("Value") 5.0 ("Value")] -> w278
              tunnel: [128.0 ("Value") 0.0 ("Value") 0.0 ("Value")] -> w277
              tunnel: [64.0 ("Value") 0.5 ("Value") 1.0 ("Value")] -> w276
              frame "PWM" {
              }
              frame "Motor", Default {
              }
              frame "Analog Out" {
              }
            }
            n138 = property on="Motor" class="Clust (strict)"("Visible"=TRUE) -> ()  [unwired: 2 in, 2 out]
            n139 = property on="Value" class="Slide (strict)"("Value"=w277, "Scale.Minimum"=w279, "Scale.Maximum"=w278, "Scale.Increment"=w276) -> ()  [unwired: 2 in, 2 out]
            n140 = property on="On/Off" class="Bool (strict)"("Visible"=w281) -> ()  [unwired: 2 in, 2 out]
            n141 = property on="Test Slider" class="Slide (strict)"("Visible"=w281) -> ()  [unwired: 2 in, 2 out]
            n142 = property on="Test Ring" class="Ring (strict)"("Visible"=w281) -> ()  [unwired: 2 in, 2 out]
            n143 = property on="Rev/Fwd" class="Clust (strict)"("Visible"=w281) -> ()  [unwired: 2 in, 2 out]
          }
          frame "Servo" {
            w297 = FALSE ("Visible")
            n144 = call <vilib>:"NT Read Number.vi"("Name"=w299) -> ("Numeric"=w298:dbl)  [unwired: 9 in, 1 out]
            n145 = property on="Test Slider" class="Slide (strict)"("Visible"=TRUE, "Scale.Maximum"=170.0 ("Scale.Range:Maximum")) -> ()  [unwired: 2 in, 2 out]
            n146 = local write "Test Slider"(w298) -> ()
            n147 = property on="Motor" class="Clust (strict)"("Visible"=w297) -> ()  [unwired: 2 in, 2 out]
            n148 = property on="Rev/Fwd" class="Clust (strict)"("Visible"=w297) -> ()  [unwired: 2 in, 2 out]
            n149 = property on="On/Off" class="Bool (strict)"("Visible"=w297) -> ()  [unwired: 2 in, 2 out]
            n150 = property on="Test Ring" class="Ring (strict)"("Visible"=w297) -> ()  [unwired: 2 in, 2 out]
          }
          frame "Relay", "Solenoid" {
            w300 = FALSE ("Visible")
            n151 = property on="Motor" class="Clust (strict)"("Visible"=w300) -> ()  [unwired: 2 in, 2 out]
            n152 = property on="Test Slider" class="Slide (strict)"("Visible"=w300) -> ()  [unwired: 2 in, 2 out]
            n153 = Search and Replace String(input string=w301, search string="/Value  **", replace string="/Direction") -> (result string=w307:string)  [unwired: 5 in, 3 out]
            n154 = property on="Test Ring" class="Ring (strict)"("Visible"=w300) -> ()  [unwired: 2 in, 2 out]
            n155 = call <vilib>:"NT Read String.vi"("Name"=w307) -> ("String"=w305:string)  [unwired: 9 in, 1 out]
            n156 = Equal?(x="Both directions", y=w305) -> (x = y?=w303:bool)
            n157 = Not(x=w303) -> (.not. x?=w304:bool)
            n158 = property on="Rev/Fwd" class="Clust (strict)"("Visible"=w303) -> ()  [unwired: 2 in, 2 out]
            n159 = property on="On/Off" class="Bool (strict)"("Visible"=w304, "Caption.Text"=w302) -> ()  [unwired: 2 in, 2 out]
          }
          frame "Compressor", "Digital Out" {
            w310 = FALSE ("Visible")
            # "Get direction and finish"
            n160 = property on="Motor" class="Clust (strict)"("Visible"=w310) -> ()  [unwired: 2 in, 2 out]
            n161 = property on="Test Slider" class="Slide (strict)"("Visible"=w310) -> ()  [unwired: 2 in, 2 out]
            n162 = property on="Test Ring" class="Ring (strict)"("Visible"=w310) -> ()  [unwired: 2 in, 2 out]
            n163 = property on="On/Off" class="Bool (strict)"("Visible"=TRUE, "Caption.Text"=w311) -> ()  [unwired: 2 in, 2 out]
            n164 = property on="Rev/Fwd" class="Clust (strict)"("Visible"=FALSE) -> ()  [unwired: 2 in, 2 out]
          }
          frame "Camera" {
            n165 = call <vilib>:"Get Last Path Segment.vi"("String in"=w318) -> ("String out"=w319:string)  [unwired: 10 in]
            n166 = property on="On/Off" class="Bool (strict)"("Visible"=FALSE) -> ()  [unwired: 2 in, 2 out]
            n167 = property on="Motor" class="Clust (strict)"("Visible"=FALSE) -> ()  [unwired: 2 in, 2 out]
            n168 = property on="Rev/Fwd" class="Clust (strict)"("Visible"=FALSE) -> ()  [unwired: 2 in, 2 out]
            n169 = case shown="\"White Balance  **\"" w319 {
              tunnel: w318 -> [w325 w334 w343 w352 w361 _ w367]
              tunnel: w317 -> [w323 w331 w340 w349 w358 _ _]
              frame "Size  **" {
                n170 = Index Array(array=w323) -> (element=w322:cluster{string[]})  [unwired: 1 in]
                n171 = call <vilib>:"NT Read String.vi"("Name"=w325) -> ("String"=w324:string)  [unwired: 9 in, 1 out]
                n172 = Unbundle(w322) -> (w320:string[])
                n173 = Match First String(2:w320, 3:w324) -> (0:w321:i32)  [unwired: 1 out]
                n174 = property on="Test Ring" class="Ring (strict)"("Value"=w321, "Strings []"=w320) -> ()  [unwired: 2 in, 2 out]
                n175 = property on="Test Ring" class="Ring (strict)"("Visible"=TRUE) -> ()  [unwired: 2 in, 2 out]
                n176 = property on="Test Slider" class="Slide (strict)"("Visible"=FALSE) -> ()  [unwired: 2 in, 2 out]
              }
              frame "White Balance  **" {
                n177 = Index Array(array=w331, index=1) -> (element=w332:cluster{string[]})
                n178 = call <vilib>:"NT Read String.vi"("Name"=w334) -> ("String"=w333:string)  [unwired: 9 in, 1 out]
                n179 = Unbundle(w332) -> (w329:string[])
                n180 = Match First String(2:w329, 3:w333) -> (0:w328:i32)  [unwired: 1 out]
                n181 = property on="Test Ring" class="Ring (strict)"("Value"=w328, "Strings []"=w329) -> ()  [unwired: 2 in, 2 out]
                n182 = property on="Test Ring" class="Ring (strict)"("Visible"=TRUE) -> ()  [unwired: 2 in, 2 out]
                n183 = property on="Test Slider" class="Slide (strict)"("Visible"=FALSE) -> ()  [unwired: 2 in, 2 out]
              }
              frame "Exposure  **" {
                n184 = Index Array(array=w340, index=2) -> (element=w341:cluster{string[]})
                n185 = call <vilib>:"NT Read String.vi"("Name"=w343) -> ("String"=w342:string)  [unwired: 9 in, 1 out]
                n186 = Unbundle(w341) -> (w337:string[])
                n187 = Match First String(2:w337, 3:w342) -> (0:w338:i32)  [unwired: 1 out]
                n188 = property on="Test Ring" class="Ring (strict)"("Value"=w338, "Strings []"=w337) -> ()  [unwired: 2 in, 2 out]
                n189 = property on="Test Ring" class="Ring (strict)"("Visible"=TRUE) -> ()  [unwired: 2 in, 2 out]
                n190 = property on="Test Slider" class="Slide (strict)"("Visible"=FALSE) -> ()  [unwired: 2 in, 2 out]
              }
              frame "Exposure Priority  **" {
                n191 = Index Array(array=w349, index=3) -> (element=w350:cluster{string[]})
                n192 = call <vilib>:"NT Read String.vi"("Name"=w352) -> ("String"=w351:string)  [unwired: 9 in, 1 out]
                n193 = Unbundle(w350) -> (w346:string[])
                n194 = Match First String(2:w346, 3:w351) -> (0:w347:i32)  [unwired: 1 out]
                n195 = property on="Test Ring" class="Ring (strict)"("Value"=w347, "Strings []"=w346) -> ()  [unwired: 2 in, 2 out]
                n196 = property on="Test Ring" class="Ring (strict)"("Visible"=TRUE) -> ()  [unwired: 2 in, 2 out]
                n197 = property on="Test Slider" class="Slide (strict)"("Visible"=FALSE) -> ()  [unwired: 2 in, 2 out]
              }
              frame "Color Enable  **" {
                n198 = Index Array(array=w358, index=4) -> (element=w359:cluster{string[]})
                n199 = call <vilib>:"NT Read String.vi"("Name"=w361) -> ("String"=w360:string)  [unwired: 9 in, 1 out]
                n200 = Unbundle(w359) -> (w355:string[])
                n201 = Match First String(2:w355, 3:w360) -> (0:w356:i32)  [unwired: 1 out]
                n202 = property on="Test Ring" class="Ring (strict)"("Value"=w356, "Strings []"=w355) -> ()  [unwired: 2 in, 2 out]
                n203 = property on="Test Ring" class="Ring (strict)"("Visible"=TRUE) -> ()  [unwired: 2 in, 2 out]
                n204 = property on="Test Slider" class="Slide (strict)"("Visible"=FALSE) -> ()  [unwired: 2 in, 2 out]
              }
              frame Default {
                n205 = property on="Test Ring" class="Ring (strict)"("Visible"=FALSE) -> ()  [unwired: 2 in, 2 out]
                n206 = property on="Test Slider" class="Slide (strict)"("Visible"=FALSE) -> ()  [unwired: 2 in, 2 out]
              }
              frame "Brightness  **", "Color Level  **", "Compression  **", "FPS  **", "Sharpness  **" {
                n207 = call <vilib>:"NT Read Number.vi"("Name"=w367) -> ("Numeric"=w366:dbl)  [unwired: 9 in, 1 out]
                n208 = local write "Test Slider"(w366) -> ()
                n209 = property on="Test Slider" class="Slide (strict)"("Visible"=TRUE, "Scale.Maximum"=100.0 ("Scale.Range:Maximum")) -> ()  [unwired: 2 in, 2 out]
                n210 = property on="Test Ring" class="Ring (strict)"("Visible"=FALSE) -> ()  [unwired: 2 in, 2 out]
              }
            }
          }
        }
        n211 = property on="Progress" class="Clust (strict)"("Visible"=FALSE) -> ()  [unwired: 2 in, 2 out]
      }
      event "Test Name": Mouse Enter {
        # "Populate the ring with the list of tests"
        n212 = event-data() -> ()  [unwired: 1 in, 1 out]
        n213 = call <vilib>:"NT Read String Array.vi"("Name"="/TestMode/TestList") -> ("String Array"=w376:string[])  [unwired: 9 in, 1 out]
        n214 = Build Array (concatenate)("Select the test to run...", w376) -> (w375:string[])
        n215 = property on="Test Name" class="Ring (strict)"("Strings []"=w375) -> ()  [unwired: 2 in, 2 out]
      }
      event "Test Name": Value Change {
        w379 = FALSE ("Visible")
        # "Tell the robot the test name to run"
        n216 = event-data() -> ("NewVal"=w383:u16)  [unwired: 1 in]
        n217 = property on="Test Name" class="Ring (strict)"() -> ("Strings []"=w384:string[])  [unwired: 2 in, 2 out]
        n218 = local write "Progress"(T8 {"Test Progress"=0, "Test Progress Text"=""} ("Progress")) -> ()
        n219 = Index Array(array=w384, index=w383) -> (element=w382:string)
        n220 = call <vilib>:"NT Write String.vi"("String"=w382, "Name"="/TestMode/TestName") -> ()  [unwired: 9 in, 1 out]
        n221 = property on="Progress" class="Clust (strict)"("Visible"=TRUE) -> ()  [unwired: 2 in, 2 out]
        n222 = property on="Motor" class="Clust (strict)"("Visible"=w379) -> ()  [unwired: 2 in, 2 out]
        n223 = property on="Test Slider" class="Slide (strict)"("Visible"=w379) -> ()  [unwired: 2 in, 2 out]
        n224 = property on="On/Off" class="Bool (strict)"("Visible"=w379) -> ()  [unwired: 2 in, 2 out]
        n225 = property on="Rev/Fwd" class="Clust (strict)"("Visible"=w379) -> ()  [unwired: 2 in, 2 out]
        n226 = property on="Test Ring" class="Ring (strict)"("Visible"=w379) -> ()  [unwired: 2 in, 2 out]
      }
      event "Select Auto": Mouse Enter {
        # "Populate the combo box with the list of autonomous options"
        n227 = event-data() -> ()  [unwired: 1 in, 1 out]
        n228 = call <vilib>:"NT Read String Array.vi"("Name"="Auto List") -> ("String Array"=w386:string[])  [unwired: 9 in, 1 out]
        n229 = property on="Select Auto" class="CmbBox"("Strings[]"=w386) -> ()  [unwired: 2 in, 2 out]
      }
      event "Select Auto": Value Change {
        # "User modified the Auto Selection. Write to NT variable so robot knows."
        n230 = event-data() -> ("NewVal"=w390:string)  [unwired: 1 in]
        n231 = call <vilib>:"NT Write String.vi"("String"=w390, "Name"="Auto Selector") -> ()  [unwired: 9 in, 1 out]
      }
      event "Command Selection": Value Change {
        # "Get the params and show in table"
        n232 = event-data() -> ("NewVal"=w397:i32)  [unwired: 1 in]
        n233 = property on="Command Selection" class="MCListbox (strict)"() -> ("ItemNames"=w395:string[][])  [unwired: 2 in, 2 out]
        n234 = call <vilib>:"WPI_DashboardUpdate Command Params.vi"("NewVal"=w397, "Commands"=w395, "Param Tbl"=w396) -> ()  [unwired: 8 in, 1 out]
      }
      event "Execute Command": Value Change {
        # "Started one, Unique ID holds\nresponse"
        n235 = event-data() -> ()  [unwired: 1 in, 1 out]
        n236 = property on="Command Selection" class="MCListbox (strict)"() -> ("ItemNames"=w409:string[][])  [unwired: 2 in, 2 out]
        n237 = Index Array(array=w409, index (row)="Command Selection", index (col)=0) -> (element=w407:string)
        n238 = call <vilib>:"Invoke Commands.vi"("Command Params"="Command Params", "Function Name"=w407) -> ("Params"=w403:u8, "Started"=w402:bool)  [unwired: 7 in, 1 out]
        n239 = Array Subset(array="Command Params", length (row)=w403) -> (w404:string[][])  [unwired: 3 in]
        n240 = Select(t="Executing" ("Cmd Status"), s=w402, f="" ("Cmd Status")) -> (s? t:f=→"Cmd Status":string)
      }
      event "Command Selection": Double Click {
        n241 = event-data() -> ("Row"=w419:i32)  [unwired: 1 in]
        n242 = property on="Command Selection" class="MCListbox (strict)"() -> ("ItemNames"=w422:string[][])  [unwired: 2 in, 2 out]
        n243 = local read "Command Params"() -> (w417:string[][])
        n244 = Index Array(array=w422, index (row)=w419, index (col)=0) -> (element=w420:string)
        n245 = call <vilib>:"Invoke Commands.vi"("Command Params"=w417, "Function Name"=w420) -> ("Params"=w416:u8, "Started"=w411:bool)  [unwired: 7 in, 1 out]
        n246 = Array Subset(array=w417, length (row)=w416) -> (w415:string[][])  [unwired: 3 in]
        n247 = Select(t="Executing" ("Cmd Status"), s=w411, f="" ("Cmd Status")) -> (s? t:f=w412:string)
        n248 = local write "Cmd Status"(w412) -> ()
      }
      event "CheckList": Double Click {
        # "Shift clears all"
        # "Update symbols on the listbox"
        n249 = event-data() -> ("PlatMods.Shift"=w425:bool, "Row"=w427:i32)  [unwired: 1 in]
        n250 = case shown="True" w425 {
          tunnel: w427 -> [w431 _]
          tunnel: 1 -> [w430 _]
          frame False {
            n251 = property on="CheckList" class="LstBox (strict)"() -> ("Item Symbols"=w429:i32[])  [unwired: 2 in, 2 out]
            n252 = Replace Array Subset(array=w429, new element=w430, index=w431) -> (w428:i32[])
            n253 = property on="CheckList" class="LstBox (strict)"("Item Symbols"=w428) -> ()  [unwired: 2 in, 2 out]
          }
          frame True {
            w432 = 0 ("Top Row")
            n254 = property on="CheckList" class="LstBox (strict)"() -> ("Number of Rows"=w434:u32)  [unwired: 2 in, 2 out]
            n255 = Initialize Array(0, w434) -> (w433:i32[])
            n256 = property on="CheckList" class="LstBox (strict)"("Top Row"=w432, "Value"=w432, "Item Symbols"=w433) -> ()  [unwired: 2 in, 2 out]
          }
        }
      }
      event "CheckList": Key Down {
        # "Update symbols on the listbox\nLeft and right keys check and uncheck"
        n257 = event-data() -> ("VKey"=w439:T23)  [unwired: 1 in]
        n258 = case shown="\"Left\", \"Right\"" w439 {
          selector: w439 -> [w444 _]
          tunnel: eventvkey."Left" ("VKey") -> [w442 _]
          frame "Left", "Right" {
            n259 = Equal?(x=w442, y=w444) -> (x = y?=w443:bool)
            n260 = Select(t=0, s=w443, f=1) -> (s? t:f=w445:i32)
            n261 = property on="CheckList" class="LstBox (strict)"() -> ("Item Symbols"=w448:i32[])  [unwired: 2 in, 2 out]
            n262 = Replace Array Subset(array=w448, new element=w445, index="CheckList") -> (w447:i32[])
            n263 = property on="CheckList" class="LstBox (strict)"("Item Symbols"=w447) -> ()  [unwired: 2 in, 2 out]
          }
          frame Default {
          }
        }
      }
      event "DB Camera Config": Value Change {
        # "Show or hide the cluster of controls, store in ini file"
        n264 = event-data() -> ("NewVal"=w453:bool)  [unwired: 1 in]
        n265 = case shown="False" w453 {
          tunnel: w452 -> [w462 _]
          tunnel: [w455 w473] -> w451
          tunnel: w450 -> [w454 w473]
          frame False {
            w469 = "Camera"
            w472 = FALSE ("Visible")
            n266 = local read "Camera Settings"() -> (w461:T2)
            n267 = Index Array(array=w462) -> (element=w465:cluster{string[]})  [unwired: 1 in]
            n268 = Unbundle(w461) -> ("Frame Rate"=w460:i32, "Compression"=w459:i32, "Size"=w463:u16)
            n269 = Unbundle(w465) -> (w464:string[])
            n270 = Index Array(array=w464, index=w463) -> (element=w458:string)
            n271 = call-poly <vilib>:"Write Key.vi"("section"=w469, "value"=w458, "key"="Size", "refnum"=w454) -> ("refnum out"=w471:T21)  [unwired: 2 in, 5 out]
            n272 = call-poly <vilib>:"Write Key.vi"("section"=w469, "value"=w460, "key"="FrameRate", "refnum"=w471) -> ("refnum out"=w470:T21)  [unwired: 1 in, 6 out]
            n273 = property on="Camera Settings" class="Clust (strict)"("Visible"=w472) -> ()  [unwired: 2 in, 2 out]
            n274 = local write "DB Camera Config"(w472) -> ()
            n275 = call-poly <vilib>:"Write Key.vi"("section"=w469, "value"=w459, "key"="Compression", "refnum"=w470) -> ("refnum out"=w456:T21)  [unwired: 1 in, 6 out]
            n276 = call <vilib>:"Close Config Data.vi"("refnum"=w456) -> ("file path"=w457:path)  [unwired: 2 in, 8 out]
            n277 = call <vilib>:"Open Config Data.vi"("configuration file path"=w457) -> ("refnum"=w455:T21)  [unwired: 8 in, 2 out]
          }
          frame True {
            n278 = property on="Camera Settings" class="Clust (strict)"("Visible"=TRUE) -> ()  [unwired: 2 in, 2 out]
          }
        }
      }
      event "Camera Settings": Value Change {
        # "Update summary string when any elements of DB camera change"
        n279 = event-data() -> ("NewVal"=w487:T2)  [unwired: 1 in]
        n280 = Index Array(array=w483) -> (element=w482:cluster{string[]})  [unwired: 1 in]
        n281 = Unbundle(w487) -> ("Frame Rate"=w478:i32, "Compression"=w477:i32, "Size"=w480:u16)
        n282 = Unbundle(w482) -> (w481:string[])
        n283 = Index Array(array=w481, index=w480) -> (element=w479:string)
        n284 = Format Into String(format string="%s   %dfps   %d%%", w479, w478, w477) -> (resulting string=w484:string)  [unwired: 2 in, 1 out]
        n285 = Build Array(w484) -> (w485:string[])
        n286 = property on="DB Camera Config" class="Bool (strict)"("Strings [4]"=w485) -> ()  [unwired: 2 in, 2 out]
      }
      event "Motor.Enable": Value Change {
        # "When the test mode otor enable helper is set, update that\ntree row item's value"
        n287 = event-data() -> ("NewVal"=w494:bool)  [unwired: 1 in]
        n288 = Unbundle("Motor") -> ("Value"=w493:dbl)  [unwired: 1 out]
        n289 = Select(t=w493, s=w494, f=0.0) -> (s? t:f=w491:dbl)
        n290 = call <vilib>:"NT Write Number.vi"("Numeric"=w491, "Name"=w490) -> ()  [unwired: 9 in, 1 out]
      }
      event "Test Slider": Value Change {
        # "When the test mode slider helper is set, update that\ntree row item's value"
        n291 = event-data() -> ("NewVal"=w498:dbl)  [unwired: 1 in]
        n292 = call <vilib>:"NT Write Number.vi"("Numeric"=w498, "Name"=w499) -> ()  [unwired: 9 in, 1 out]
      }
      event "On/Off": Value Change {
        # "When the test mode on/off helper value is set, update that\ntree row item's value"
        n293 = event-data() -> ("NewVal"=w504:bool)  [unwired: 1 in]
        n294 = Boolean To (0,1)(Boolean=w504) -> (0, 1=w503:i16)
        n295 = call <vilib>:"NT Write Number.vi"("Numeric"=w503, "Name"=w502) -> ()  [unwired: 9 in, 1 out]
      }
      event "Rev/Fwd": Value Change {
        # "When the test mode helper value for relays is set, update that\ntree row item's value"
        n296 = event-data() -> ("NewVal.Forward"=w513:bool, "NewVal.Reverse"=w512:bool)  [unwired: 1 in]
        n297 = Boolean To (0,1)(Boolean=w513) -> (0, 1=w509:i16)
        n298 = Boolean To (0,1)(Boolean=w512) -> (0, 1=w511:i16)
        n299 = Negate(x=w511) -> (-x=w510:i16)
        n300 = Add(x=w509, y=w510) -> (x+y=w508:i16)
        n301 = call <vilib>:"NT Write Number.vi"("Numeric"=w508, "Name"=w507) -> ()  [unwired: 9 in, 1 out]
      }
      event "Test Ring": Value Change {
        # "When a test mode helper value is selected from the ring,\nset the tree item's variable to the string value"
        n302 = event-data() -> ("NewVal"=w518:u16)  [unwired: 1 in]
        n303 = property on="Test Ring" class="Ring (strict)"() -> ("Strings []"=w519:string[])  [unwired: 2 in, 2 out]
        n304 = Index Array(array=w519, index=w518) -> (element=w517:string)
        n305 = call <vilib>:"NT Write String.vi"("String"=w517, "Name"=w516) -> ()  [unwired: 9 in, 1 out]
      }
      event "Rec Mode": Value Change {
        # "Update globals for recording mode and path to read log from.\nClear when logging and let NetworkTables set path for vision to\nuse."
        n306 = event-data() -> ("NewVal"=w531:enum32{"Stop", "Record", "Playback"})  [unwired: 1 in]
        n307 = global write "WPI_DashboardLogging Global.vi" "Logging Filename"(path "") -> ()
        n308 = global write "WPI_DashboardLogging Global.vi" "Recording"(w531) -> ()
        n309 = case shown="\"Playback\"" w531 {
          tunnel: w530 -> [_ w533 w542]
          tunnel: [_ _ w541] -> w527
          tunnel: [_ _ w540] -> _
          tunnel: w525 -> [_ _ w538]
          tunnel: cluster{i32, i32} {-250, 170} -> [_ _ w537]
          tunnel: [_ _ T24 {"Image Size"=TRUE, "Image Type"=TRUE, "Pixel Value"=TRUE, "ROI Information"=TRUE, "Zoom Factor"=FALSE} ("Image Information Shown:All Elements")] -> w523
          tunnel: [_ _ TRUE ("Zoom Factor")] -> w522
          tunnel: w521 -> [_ _ w534]
          frame Default {
          }
          frame "Stop", "Record" {
            # "Place Window too"
            n310 = invoke class="VI" method="FP.Close"(reference=w533) -> (reference out=w532:refnum<vi>)  [unwired: 2 in, 2 out]
            n311 = invoke class="VI" method="Abort VI"(reference=w532) -> ()  [unwired: 2 in, 3 out]
          }
          frame "Playback" {
            n312 = call "Open Playback Panel.vi"("Offset"=w537, "DB VI Ref"=w538, "Playback in"=w542) -> ("Playback out"=w539:refnum<vi>)  [unwired: 8 in]
            n313 = register-events(w539, w534) -> (reference out=w541:refnum<event-registration>, error out=w540:errorcluster)  [unwired: 2 in]
          }
        }
        n314 = property on="Camera Image" class="ImageControl"("Image Information Shown"=w523, "Image Information Visible"=w522) -> ()  [unwired: 2 in, 2 out]
        n315 = call <vilib>:"WPI_DashboardNT Log FieldName Cache.vi"("Operation"=enum16{"Lookup/Add", "Index", "Clear"}."Clear") -> ()  [unwired: 8 in, 3 out]
      }
      event Panel Close {
        w544 = enum32{"Stop", "Record", "Playback"}."Stop" ("Rec Mode")
        # "Playback window has been closed, abort"
        n316 = event-data() -> ()  [unwired: 1 in, 4 out]
        n317 = local write "Rec Mode"(w544) -> ()
        n318 = global write "WPI_DashboardLogging Global.vi" "Recording"(w544) -> ()
      }
      event Panel Close {
        # "Abort playback window and ourself"
        n319 = event-data() -> ()  [unwired: 1 in, 4 out]
        n320 = invoke class="VI" method="FP.Close"(reference=w550) -> (reference out=w549:refnum<vi>)  [unwired: 2 in, 2 out]
        n321 = invoke class="VI" method="Abort VI"(reference=w549) -> (error out=w548:errorcluster)  [unwired: 2 in, 2 out]
        n322 = invoke class="VI" method="Abort VI"(error in=w548) -> ()  [unwired: 2 in, 3 out]
      }
      event User Event {
        n323 = event-data() -> ("IDs"=w558:cluster{"RPC field ID":u16, "Unique ID":u16}, "String"=w557:string)  [unwired: 1 in]
        n324 = Bundle("IDs"=w558, "String"=w557) -> (w556:T10)  [unwired: 1 in]
        n325 = call <vilib>:"Retrieve RPC Response.vi"("RPC Response"=w556) -> ("Output"=w553:string[][])  [unwired: 10 in]
        n326 = Build Array (concatenate)(w551, w553) -> (w552:string[][])
        n327 = local write "Command Params"(w552) -> ()
        n328 = local write "Cmd Status"("" ("Cmd Status")) -> ()
      }
      event "Vision": Value Change {
        # "Enable/Disable Compression slider.\nHW USB is hard-coded into the camera"
        n329 = event-data() -> ("NewVal"=w565:u16)  [unwired: 1 in]
        n330 = Equal?(x=w565, y=u32 2 ("milliseconds to wait")) -> (x = y?=w563:bool)
        n331 = Select(t=T25."Disabled and Grayed Out" ("Disabled"), s=w563, f=T25."Enabled" ("Disabled")) -> (s? t:f=w560:T25)
        n332 = property on="Compression" class="Slide (strict)"("DisabledEnum"=w560) -> ()  [unwired: 2 in, 2 out]
      }
      event "Tree": Double Click {
        n333 = event-data() -> ("PlatMods"=w570:T28, "Tag"=w569:string)  [unwired: 1 in]
        n334 = Unbundle(w570) -> ("Shift"=w568:bool)  [unwired: 4 out]
        n335 = Not(x=w568) -> (.not. x?=w567:bool)
        n336 = call <vilib>:"NT Update Persistence.vi"("Persistence"=w567, "Name"=w569) -> ()  [unwired: 9 in, 1 out]
      }
    }
  }
  n337 = while {
    tunnel: w47 -> [w574]
    i -> [w577]
    stop <- FALSE stop-if-true
    n338 = Wait (ms)(milliseconds to wait=u32 100) -> ()  [unwired: 1 out]
    n339 = case shown="\"Playback\"" "Rec Mode" {
      tunnel: w577 -> [_ _ w592]
      tunnel: [u32 2829099 ("Base Color") u32 11141120 ("Target Color") w581] -> w573
      frame "Stop", Default {
        # "Reset the color, extra updates don't cost much"
      }
      frame "Record" {
      }
      frame "Playback" {
        # "Playback"
        n340 = Quotient & Remainder(x=w592, y=u32 50 ("milliseconds to wait")) -> (x-y*floor(x/y)=w588:u32)  [unwired: 1 out]
        n341 = Divide(x=w588, y=u32 50 ("milliseconds to wait")) -> (x/y=w585:dbl)
        n342 = Multiply(x=6.283185307179586, y=w585) -> (x*y=w590:dbl)
        n343 = Sine(x=w590) -> (sin(x)=w589:dbl)
        n344 = Absolute Value(x=w589) -> (abs(x)=w582:dbl)
        n345 = call "Interpolate RGB Color.vi"("Proportion"=w582, "Target Color"=u32 30976, "Base Color"=u32 2829099) -> ("Result Color"=w581:u32)  [unwired: 8 in]
      }
    }
    n346 = property class="Pane"(reference=w574, "PaneColor"=w573) -> ()  [unwired: 1 in, 2 out]
  }
  n347 = local write "Dashboard Tab"(T1."I/O" ("Dashboard Tab")) -> ()
  n348 = property on="On/Off" class="Bool (strict)"("Visible"=w15) -> ()  [unwired: 2 in, 2 out]
  n349 = property on="Motor" class="Clust (strict)"("Visible"=w15) -> ()  [unwired: 2 in, 2 out]
  n350 = property on="Progress" class="Clust (strict)"("Visible"=w15) -> ()  [unwired: 2 in, 2 out]
  n351 = property on="Test Ring" class="Ring (strict)"("Visible"=w15) -> ()  [unwired: 2 in, 2 out]
  n352 = property on="Rev/Fwd" class="Clust (strict)"("Visible"=w15) -> ()  [unwired: 2 in, 2 out]
  n353 = property on="Camera Settings" class="Clust (strict)"("Visible"=w15) -> ()  [unwired: 2 in, 2 out]
  n354 = local write "DB Camera Config"(w15) -> ()
  n355 = local write "Command Params"(string[][] [] ("Command Params")) -> ()
  n356 = global write "WPI_DashboardLogging Global.vi" "Recording"(w41) -> ()
  n357 = local write "Rec Mode"(w41) -> ()
  n358 = while {
    tunnel: u16 1741 ("timeout ms (25000)") -> [w594]
    stop <- FALSE stop-if-true
    n359 = TCP Create Listener(10:w594) -> (0:w593:errorcluster, 3:w595:refnum<k5>)  [unwired: 4 in, 1 out]
    n360 = case shown="No Error" w593 {
      selector: w593 -> [w597 _]
      tunnel: w595 -> [w598 _]
      frame No Error {
        n361 = while {
          tunnel: w598 -> [w601]
          tunnel: w597 -> [w600]
          stop <- FALSE stop-if-true
          n362 = TCP Wait On Listener(8:w600, 11:w601) -> (0:w602:errorcluster, 4:w603:refnum<k5>)  [unwired: 2 in, 3 out]
          n363 = local write "TCP"(w603) -> ()
          n364 = case shown="No Error" w602 {
            frame No Error {
            }
            frame Error {
              n365 = Wait (ms)(milliseconds to wait=u32 1000) -> ()  [unwired: 1 out]
            }
          }
        }
      }
      frame Error {
        n366 = Wait (ms)(milliseconds to wait=u32 1000) -> ()  [unwired: 1 out]
      }
    }
  }
  n367 = local write "Command Selection"(u16 0 ("milliseconds to wait")) -> ()
